vi "Info.vi"() -> (0 "error out":errorcluster, 2 "LibraryName":string, 3 "VI Name":string)   [LabVIEW 2011, in "NBC.lvlib"]
uses:
  NBC.lvlib
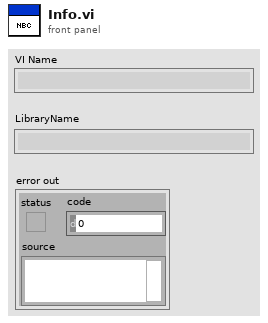
[diagram p1: front panel]
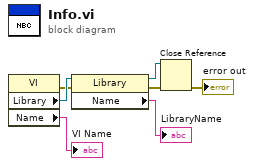
[diagram p0: block diagram]
diagram:
  n1 = property class="VI"() -> (error out=w6:errorcluster, "Library"=w7:refnum<vi>, "Name"=→"VI Name":string)  [unwired: 2 in, 1 out]
  n2 = property class="Library"(reference=w7, error in=w6) -> (reference out=w2:refnum<vi>, error out=w3:errorcluster, "Name"=→"LibraryName":string)
  n3 = Close Reference(reference=w2, error in (no error)=w3) -> (error out=→"error out":errorcluster)
